vi "ask.vi"() -> ()   [LabVIEW 2024]
panel:
  out "element":cluster{dbl, dbl}
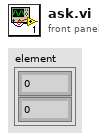
[diagram p1: front panel]
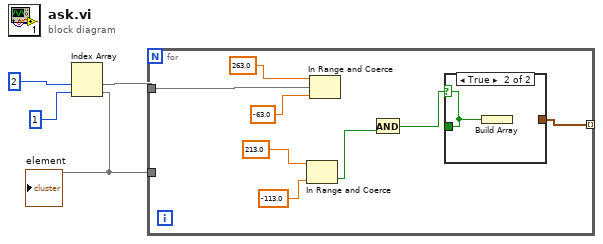
[diagram p0: block diagram]
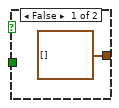
[diagram p2: hidden frame]
diagram:
  n1 = Index Array(index #1=2 ("index"), index #2=1 ("index")) -> (array=w5:cluster{dbl, dbl}[], element #1=w4, element #2=w3)
  "element" <- w3
  n2 = for {
    tunnel: w4 -> [w9]
    tunnel: w3 -> [_]
    tunnel: [w8] -> _ mode=indexing
    n3 = In Range and Coerce(upper limit=213.0, lower limit=-113.0) -> (In Range?=w6:bool)  [unwired: 1 in, 1 out]
    n4 = In Range and Coerce(upper limit=263.0, x=w9, lower limit=-63.0) -> ()  [unwired: 2 out]
    n5 = And(y=w6) -> (x .and. y?=w7:bool)  [unwired: 1 in]
    n6 = case shown="True" w7 {
      selector: w7 -> [_ w15]
      tunnel: [_ w15] -> _
      tunnel: [cluster{i32, i32}[] [] _] -> w8
      frame False {
      }
      frame True {
        n7 = Build Array(w15) -> ()  [unwired: 1 out]
      }
    }
  }
